vi "CAN Log.vi"(4 "TX/RX?":enum16{"Tx", "Rx"}(ring), 5 "Log?":bool, 6 "Action":enum16{"Update Table", "Clear Table"}(ring), 7 "CAN frame":T1 {"payload" format="%x"; "timestamp" format="%<%.7X\n%x>T"; "type" items=["CAN Data"=0, "CAN Remote"=1, "CAN Bus Error"=2, "CAN 2.0 Data"=8, "CAN FD Data"=16, "CAN FD+BRS Data"=24, "J1939 Data"=192, "Delay"=224, "Log Trigger"=225, "Start Trigger"=226]; "identifier" format="%x"}, 8 "error in (no error)":errorcluster, 9 "Socket No":i16, 10 "Hexadecimal?":bool=TRUE, 11 "CAN View Table":refnum<vi>) -> (0 "error out":errorcluster)   [LabVIEW 2023, in "LTT_TeststandSteptypes.lvlib"]
uses:
  LTT_TeststandSteptypes.lvlib
  HardwareAbstractionLayer_LVOOP/CAN/CAN Lib/Control/CAN Table.ctl
  <vilib>/xnet/xnet.llb/XNET Frame CAN.ctl
  <vilib>/xnet/xnet.llb/XNET Frame Type CAN.ctl
  HardwareAbstractionLayer_LVOOP/CAN/CAN Lib/Control/CAN Log Data.ctl
  Control/CAN FGV State.ctl
  HardwareAbstractionLayer_LVOOP/Report/Report_class/Control/Action FGV.ctl
  <vilib>/Utility/error.llb/Trim Whitespace One-Sided.vi
  HardwareAbstractionLayer_LVOOP/CAN/CAN Lib/CAN HAL Lib.lvlib
  HardwareAbstractionLayer_LVOOP/Report/Report_class/Report.lvclass
panel:
  out "appended array":string[](array[string])
  out "Output Array":string[][](array[string])
  in  "CAN View Table":T3=-1
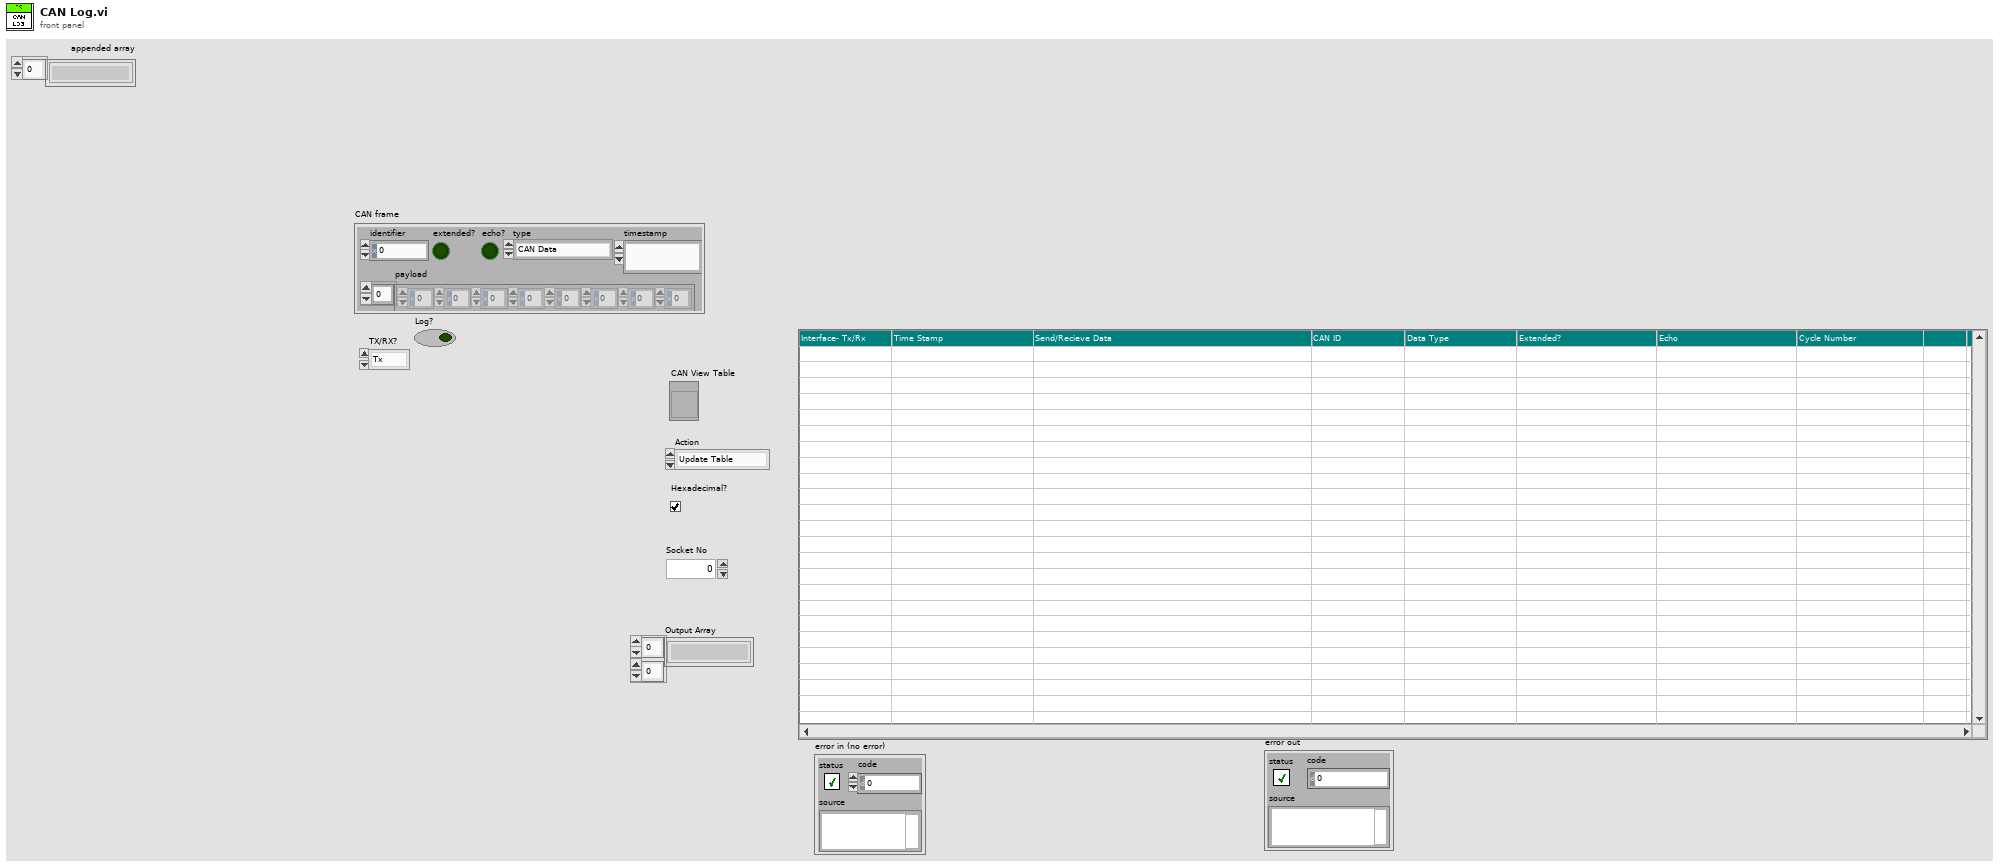
[diagram p1: front panel]
types:
  T1 = typedef "XNET Frame CAN.ctl" = cluster{"timestamp":timestamp, "payload":u8[], "identifier":u32, "type":T2, "extended?":bool, "echo?":bool}
  T2 = typedef "XNET Frame Type CAN.ctl" = u8
  T3 = typedef "HardwareAbstractionLayer_LVOOP.lvlib/CAN HAL Lib.lvlib/CAN Table.ctl" = i32
  T4 = typedef "HardwareAbstractionLayer_LVOOP.lvlib/CAN HAL Lib.lvlib/CAN Log Data.ctl" = cluster{"Data":T1[], "TX/RX?":enum16{"Tx", "Rx"}, "Interface":string}
  T5 = typedef "LTT_TeststandSteptypes.lvlib/CAN FGV State.ctl" = enum16{"Init", "Get", "Set"}
  T6 = typedef "HardwareAbstractionLayer_LVOOP.lvlib/Report.lvclass/Action FGV.ctl" = enum16{"Init", "Set Project Name", "Set Product Name", "Set Product Varient", "Set Test Name", "Set Test Phase", "Set Test Description", "Set Temp Chamber Name", "Set Cycle Duration", "Set Current Cycle Number", "Set Schema", "Set Total No Of Cycle", "Set Current Test Mode", "Set All Data", "Get All Data"}
  T7 = typedef "HardwareAbstractionLayer_LVOOP.lvlib/Report.lvclass/Result FGV Data.ctl" = cluster{"Project Name":string, "Product Name":string, "Product Varient":string, "Test Name":string, "Test Phase":string, "Test Description":string, "Temp Chamber Name":string, "Schema":string, "Total No of Cycles":u32, "Current Cycle Number":u32, "Cycle Duration":u32, "Current Test Mode":string}
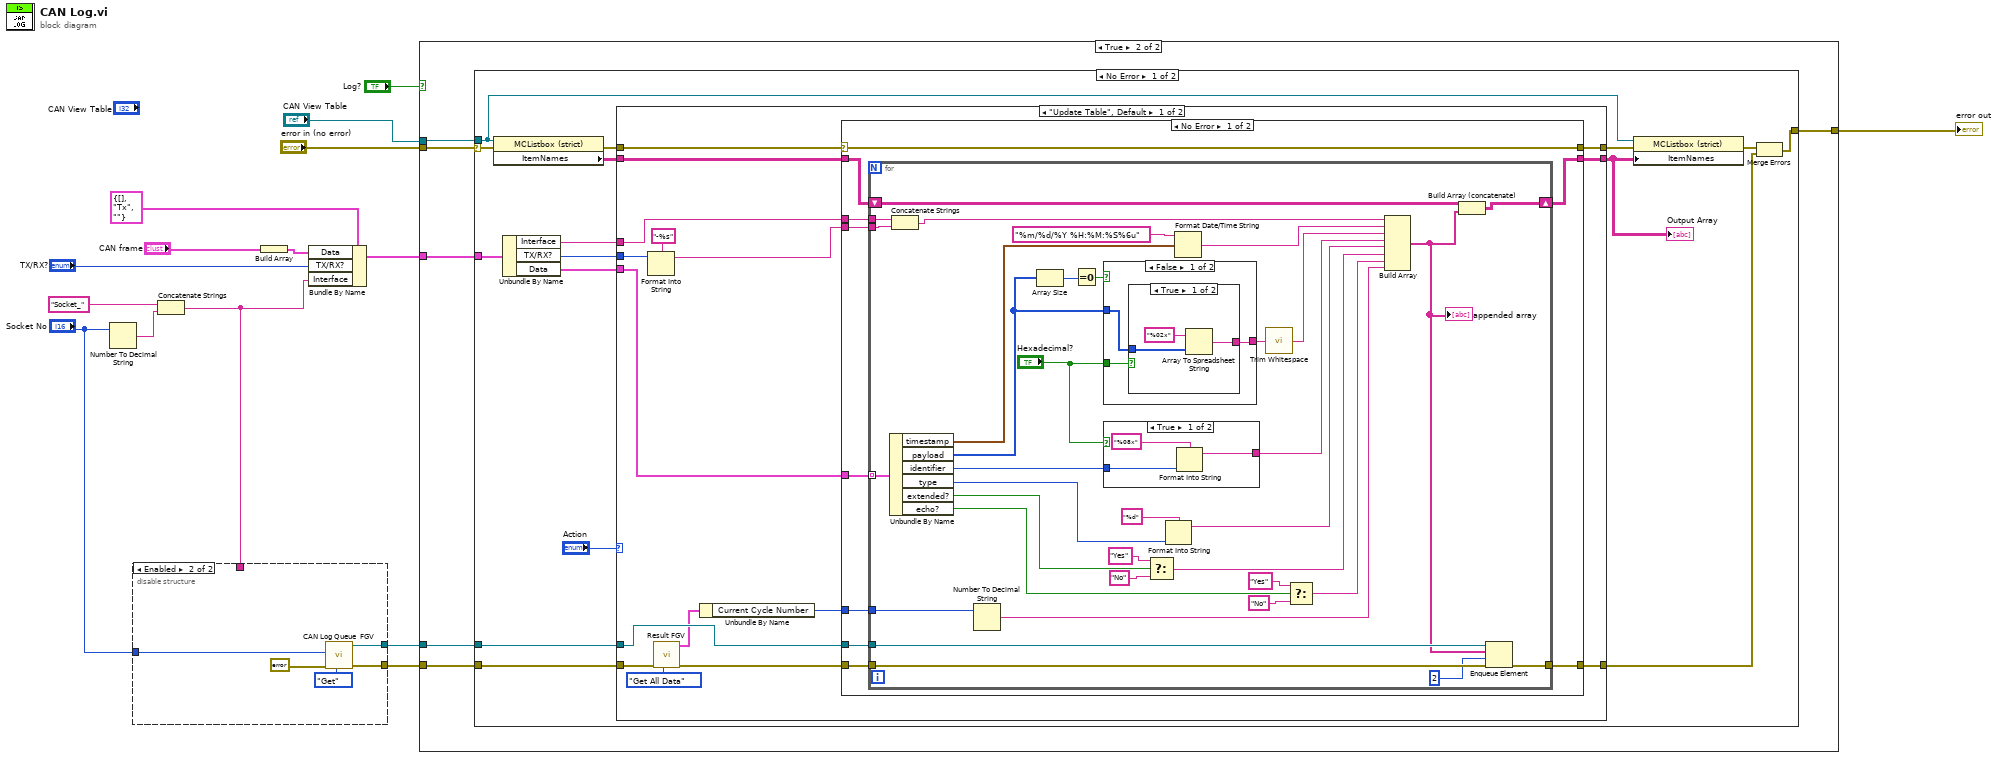
[diagram p0: block diagram]
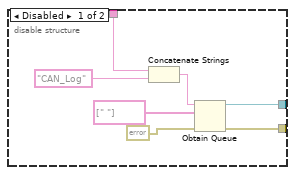
[diagram p2: hidden frame]
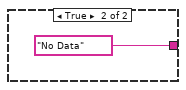
[diagram p5: hidden frame]
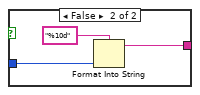
[diagram p6: hidden frame]
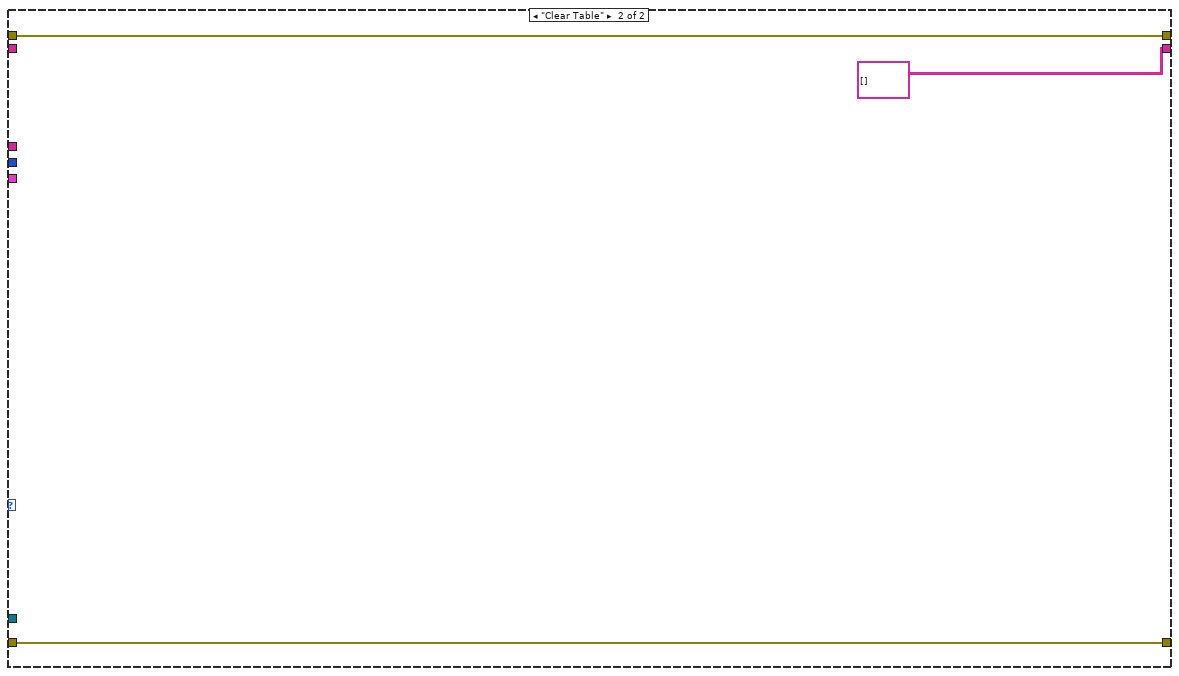
[diagram p8: hidden frame]
diagram:
  n1 = Number To Decimal String(number="Socket No") -> (decimal integer string=w12:string)  [unwired: 1 in]
  n2 = Concatenate Strings("Socket_" ("name (unnamed)"), w12) -> (w4:string)
  n3 = disable-structure shown="Enabled" {
    disable-tunnel: w4 -> [w22 _]
    disable-tunnel: [w18 w26] -> w3
    disable-tunnel: [w16 w27] -> w2
    disable-tunnel: "Socket No" -> [_ w23]
    frame Disabled {
      n4 = Concatenate Strings(w22, "CAN_Log" ("string")) -> (w21:string)
      n5 = Obtain Queue(name (unnamed)=w21, element data type=string[] [" "] ("appended array"), error in (no error)=errorcluster {"status"=FALSE, "code"=0, "source"=""}) -> (queue out=w16:refnum<queue>, error out=w18:errorcluster)  [unwired: 2 in, 1 out]
    }
    frame Enabled {
      n6 = call "CAN Log Queue  FGV.vi"("CAN FGV State"=CAN_FGV_State."Get", "error in"=errorcluster {"status"=FALSE, "code"=0, "source"=""}, "Current Scoket"=w23) -> ("error out"=w26:errorcluster, "Log queue out"=w27:refnum<queue>)  [unwired: 7 in]
    }
  }
  n7 = Build Array("CAN frame") -> (w6:T1[])
  n8 = Bundle By Name(cluster=T4 {"Data"=[], "TX/RX?"=enum."Tx", "Interface"=""} ("CAN Data"), "Data"=w6, "TX/RX?"="TX/RX?", "Interface"=w4) -> (w10:T4)
  n9 = case shown="True" "Log?" {
    tunnel: "CAN View Table" -> [_ w34]
    tunnel: [w28 w33] -> w13
    tunnel: w10 -> [_ w32]
    tunnel: "error in (no error)" -> [w28 w31]
    tunnel: w3 -> [_ w30]
    tunnel: w2 -> [_ w29]
    frame False {
    }
    frame True {
      n10 = case shown="No Error" w31 {
        selector: w31 -> [w43 w134]
        tunnel: w32 -> [w46 _]
        tunnel: w34 -> [w41 _]
        tunnel: [w36 w134] -> w33
        tunnel: w30 -> [w38 _]
        tunnel: w29 -> [w37 _]
        frame No Error {
          n11 = property class="MCListbox (strict)"(reference=w41, error in=w43) -> (error out=w49:errorcluster, "ItemNames"=w50:string[][])  [unwired: 1 out]
          n12 = Unbundle By Name(w46) -> ("Interface"=w44:string, "TX/RX?"=w42:enum16{"Tx", "Rx"}, "Data"=w45:T1[])
          n13 = case shown="\"Update Table\", Default" "Action" {
            tunnel: w45 -> [w66 _]
            tunnel: w50 -> [w65 _]
            tunnel: [w64 string[][] [] ("Value")] -> w47
            tunnel: [w63 w132] -> w40
            tunnel: w49 -> [w62 w132]
            tunnel: w44 -> [w61 _]
            tunnel: w42 -> [w60 _]
            tunnel: w38 -> [w55 w131]
            tunnel: w37 -> [w57 _]
            tunnel: [w56 w131] -> w35
            frame "Update Table", Default {
              n14 = Format Into String(format string="-%s", w60) -> (resulting string=w58:string)  [unwired: 2 in, 1 out]
              n15 = call "Result FGV.vi"("Action(Get All Data)"=Action_FGV."Get All Data", "error in"=w55) -> ("error out"=w54:errorcluster, "Result FGV Data Out"=w52:T7)  [unwired: 8 in]
              n16 = Unbundle By Name(w52) -> ("Current Cycle Number"=w51:u32)
              n17 = case shown="No Error" w62 {
                selector: w62 -> [w76 w130]
                tunnel: [w76 w130] -> w63
                tunnel: w66 -> [w75 _]
                tunnel: w65 -> [w74 w129]
                tunnel: [w73 w129] -> w64
                tunnel: w61 -> [w72 _]
                tunnel: w58 -> [w71 _]
                tunnel: w57 -> [w70 _]
                tunnel: w54 -> [w69 w128]
                tunnel: [w68 w128] -> w56
                tunnel: w51 -> [w67 _]
                frame No Error {
                  n18 = for {
                    tunnel: w75 -> [w111] mode=indexing
                    shift-right: [w104] -> w73
                    shift-left: w74 -> [w103]
                    tunnel: w72 -> [w98]
                    tunnel: w71 -> [w85]
                    tunnel: w70 -> [w83]
                    tunnel: w69 -> [w82]
                    tunnel: [w80] -> w68
                    tunnel: w67 -> [w78]
                    n19 = Unbundle By Name(w111) -> ("timestamp"=w110:timestamp, "payload"=w99:u8[], "identifier"=w101:u32, "type"=w96:T2, "extended?"=w91:bool, "echo?"=w87:bool)
                    n20 = Concatenate Strings(w98, w85) -> (w86:string)
                    n21 = Number To Decimal String(number=w78) -> (decimal integer string=w77:string)  [unwired: 1 in]
                    n22 = Array Size(array=w99) -> (size(s)=w108:i32)
                    n23 = Equal To 0?(x=w108) -> (x = 0?=w107:bool)
                    n24 = case shown="False" w107 {
                      tunnel: [w112 "No Data"] -> w105
                      tunnel: w99 -> [w114 _]
                      tunnel: "Hexadecimal?" -> [w113 _]
                      frame False {
                        n25 = case shown="True" w113 {
                          tunnel: w114 -> [w116 w119]
                          tunnel: [w115 w118] -> w112
                          frame True {
                            n26 = Array To Spreadsheet String(array=w116, 3:"%02x" ("format string")) -> (spreadsheet string=w115:string)  [unwired: 1 in]
                          }
                          frame False {
                            n27 = Array To Spreadsheet String(array=w119, 3:"%3d" ("format string")) -> (spreadsheet string=w118:string)  [unwired: 1 in]
                          }
                        }
                      }
                      frame True {
                      }
                    }
                    n28 = case shown="True" "Hexadecimal?" {
                      tunnel: w101 -> [w123 w126]
                      tunnel: [w122 w125] -> w109
                      frame True {
                        n29 = Format Into String(format string="%08x", w123) -> (resulting string=w122:string)  [unwired: 2 in, 1 out]
                      }
                      frame False {
                        n30 = Format Into String(format string="%10d", w126) -> (resulting string=w125:string)  [unwired: 2 in, 1 out]
                      }
                    }
                    n31 = Select(t="Yes", s=w91, f="No") -> (s? t:f=w92:string)
                    n32 = Format Into String(format string="%d", w96) -> (resulting string=w95:string)  [unwired: 2 in, 1 out]
                    n33 = Format Date/Time String(time format string (%c)="%m/%d/%Y %H:%M:%S%6u", seconds (now)=w110) -> (date/time string=w100:string)  [unwired: 1 in]
                    n34 = call <vilib>:"Trim Whitespace.vi"("string"=w105) -> ("trimmed string"=w102:string)  [unwired: 1 in]
                    n35 = Select(t="Yes", s=w87, f="No") -> (s? t:f=w88:string)
                    n36 = Build Array(w86, w100, w102, w109, w95, w92, w88, w77) -> (w81:string[])
                    "appended array" <- w81
                    n37 = Build Array (concatenate)(w103, w81) -> (w104:string[][])
                    n38 = Enqueue Element(queue=w83, element=w81, timeout in ms (-1)=2, error in (no error)=w82) -> (error out=w80:errorcluster)  [unwired: 2 out]
                  }
                }
                frame Error {
                }
              }
            }
            frame "Clear Table" {
            }
          }
          "Output Array" <- w47
          n39 = property class="MCListbox (strict)"(reference=w41, error in=w40, "ItemNames"=w47) -> (error out=w39:errorcluster)  [unwired: 1 out]
          n40 = Merge Errors(w39, w35) -> (w36:errorcluster)
        }
        frame Error {
        }
      }
    }
  }
  "error out" <- w13
